vi "write commands.vi"(8 "error in":errorcluster, 9 "Timeout (ms)":i32=-1, 10 "commands":T1[](array[typedef]), 11 "profibus reference":T3) -> (0 "error out":errorcluster, 3 "profibus reference out":T3)   [LabVIEW 2013, in "dynamic profibus.lvlib"]
uses:
  dynamic profibus.lvlib
  fpga reference.ctl
  full command.ctl
  profibus master action.ctl
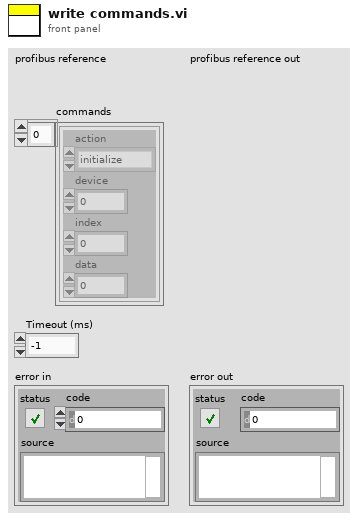
[diagram p1: front panel]
types:
  T1 = typedef "dynamic profibus.lvlib/full command.ctl" = cluster{"action":T2, "device":u8, "index":u8, "data":u8}
  T2 = typedef "dynamic profibus.lvlib/profibus master action.ctl" = enum8{"initialize", "uninitialize", "stop", "get input", "get input size", "set output", "get output size", "get diagnostic", "transfer data", "transfer diagnostics"}
  T3 = typedef "dynamic profibus.lvlib/fpga reference.ctl" = refnum<k20>
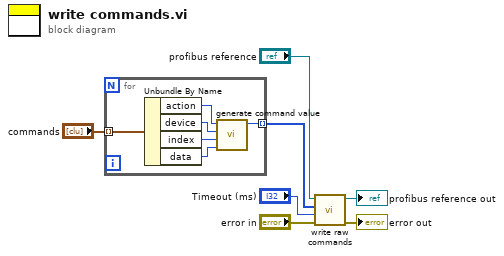
[diagram p0: block diagram]
diagram:
  n1 = for {
    tunnel: [w13] -> w2 mode=indexing
    tunnel: "commands" -> [w12] mode=indexing
    n2 = Unbundle By Name(w12) -> ("action"=w8:T2, "device"=w9:u8, "index"=w11:u8, "data"=w10:u8)
    n3 = call "generate command value.vi"("data"=w10, "index"=w11, "device"=w9, "action"=w8) -> ("Element"=w13:u32)  [unwired: 7 in]
  }
  n4 = call "write raw commands.vi"("error in"="error in", "Timeout (ms)"="Timeout (ms)", "Data"=w2, "profibus reference"="profibus reference") -> ("error out"=→"error out":errorcluster, "profibus reference out"=→"profibus reference out":T3)  [unwired: 6 in]
